vi "arreglos bidi2.vi"() -> ()   [LabVIEW 2011]
panel:
  in  "salir":bool
  in  "Sumarcolumnas":bool
  in  "Rellenar":bool
  out "Array":dbl[][](array[numeric])
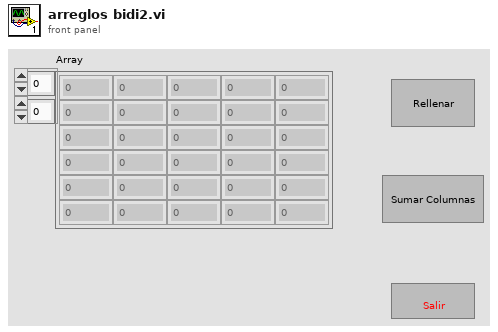
[diagram p1: front panel]
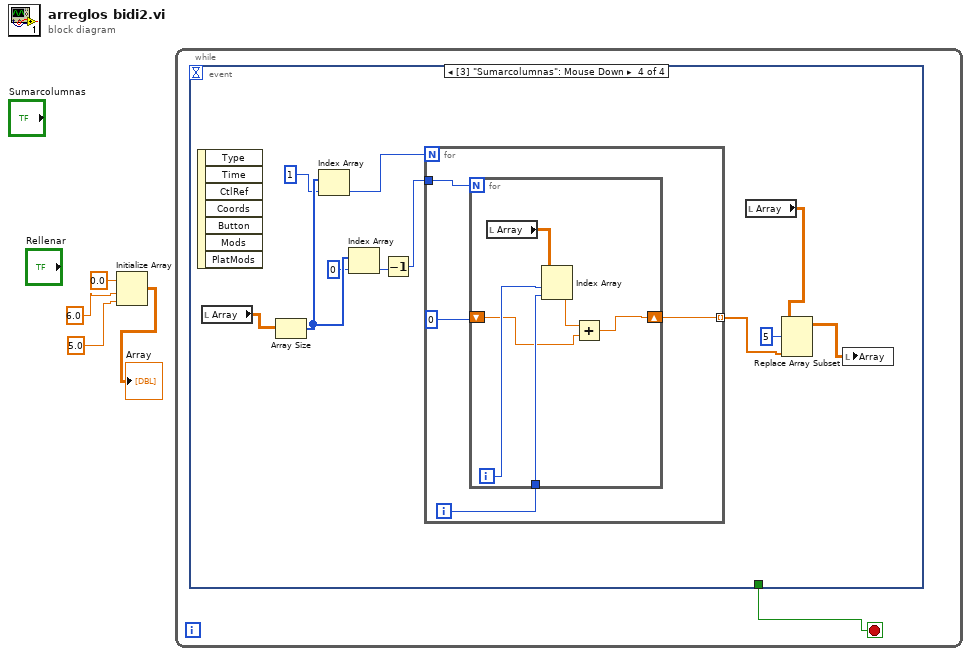
[diagram p0: block diagram]
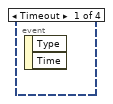
[diagram p2: hidden frame]
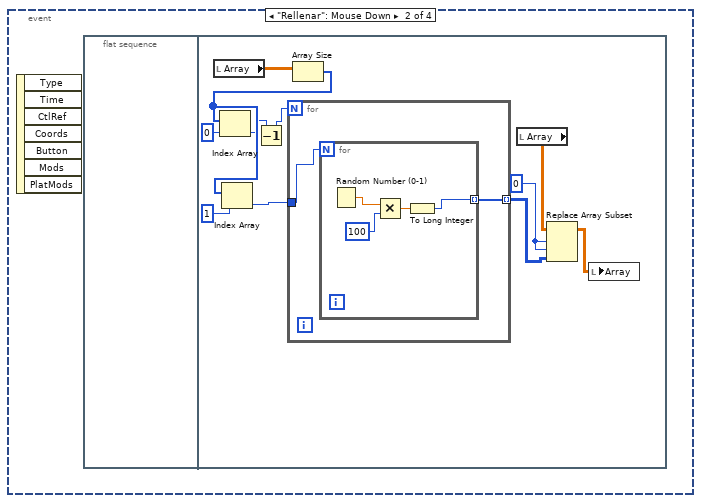
[diagram p3: hidden frame]
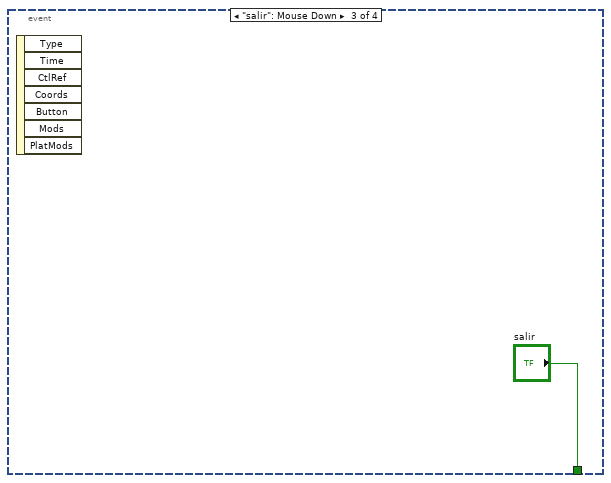
[diagram p4: hidden frame]
diagram:
  n1 = Initialize Array "Initialize Array"(0.0 ("element"), 6.0 ("element"), 5.0 ("element")) -> (→"Array":dbl[][])
  n2 = while {
    stop <- w5 stop-if-true
    n3 = event shown="[3] \"Sumarcolumnas\": Mouse Down" {
      selector: _ -> [_ _ _ _]
      dyn-events: _ -> [_ _ _ _]
      timeout: _ -> [_ _ _ _]
      tunnel: [_ _ "salir" _] -> w5
      event Timeout {
        n4 = event-data() -> ()  [unwired: 1 in, 2 out]
      }
      event "Rellenar": Mouse Down {
        n5 = event-data() -> ()  [unwired: 1 in, 7 out]
        n6 = flat-sequence {
          frame #0 {
          }
          frame #1 {
            w6 = 0 ("index")
            n7 = local read "Array"() -> (w16:dbl[][])
            n8 = Array Size(array=w16) -> (size(s)=w14:i32[])
            n9 = Index Array "Index Array"(array=w14, index=0) -> (element=w11:i32)
            n10 = Index Array "Index Array"(array=w14, index=1) -> (element=w12:i32)
            n11 = Decrement(x=w11) -> (x-1=w10:i32)
            n12 = for {
              N: w10 -> [_]
              tunnel: w12 -> [w18]
              tunnel: [w17] -> w7 mode=indexing
              n13 = for {
                N: w18 -> [_]
                tunnel: [w19] -> w17 mode=indexing
                n14 = Random Number (0-1)() -> (number: 0 to 1=w22:dbl)
                n15 = Multiply(x=w22, y=100) -> (x*y=w20:dbl)
                n16 = To Long Integer(number=w20) -> (32bit integer=w19:i32)
              }
            }
            n17 = local read "Array"() -> (w8:dbl[][])
            n18 = Replace Array Subset "Replace Array Subset"(array=w8, new element=w7, index (row)=w6, index (col)=w6) -> (w9:dbl[][])
            n19 = local write "Array"(w9) -> ()
          }
        }
      }
      event "salir": Mouse Down {
        n20 = event-data() -> ()  [unwired: 1 in, 7 out]
      }
      event "Sumarcolumnas": Mouse Down {
        n21 = event-data() -> ()  [unwired: 1 in, 7 out]
        n22 = local read "Array"() -> (w34:dbl[][])
        n23 = Array Size(array=w34) -> (size(s)=w33:i32[])
        n24 = Index Array "Index Array"(array=w33, index=1) -> (element=w32:i32)
        n25 = Index Array "Index Array"(array=w33, index=0) -> (element=w30:i32)
        n26 = Decrement(x=w30) -> (x-1=w29:i32)
        n27 = for {
          N: w32 -> [_]
          tunnel: w29 -> [w38]
          tunnel: [w35] -> w25 mode=indexing
          i -> [w37]
          n28 = for {
            N: w38 -> [_]
            tunnel: w37 -> [w42]
            shift-right: [w39] -> w35
            shift-left: 0 ("index") -> [w40]
            i -> [w43]
            n29 = local read "Array"() -> (w44:dbl[][])
            n30 = Index Array "Index Array"(array=w44, index (row)=w43, index (col)=w42) -> (element=w41:dbl)
            n31 = Add(x=w41, y=w40) -> (x+y=w39:dbl)
          }
        }
        n32 = local read "Array"() -> (w27:dbl[][])
        n33 = Replace Array Subset "Replace Array Subset"(array=w27, new element=w25, index (row)=5) -> (w26:dbl[][])  [unwired: 1 in]
        n34 = local write "Array"(w26) -> ()
      }
    }
  }
